vi "诊断标定3 - 副本.vi"(8 "CAN端口":u16(ring), 9 "设备索引号":u16(ring), 10 "CAN卡类型":u32(ring)=21) -> ()   [LabVIEW 2013] (continued)
            n1767 = property on="最小允许单体电压" class="DigNum (严格)"("Disabled"=w2295) -> ()  [unwired: 2 in, 2 out]
            n1768 = property on="电流步长" class="DigNum (严格)"("Disabled"=w2295) -> ()  [unwired: 2 in, 2 out]
            n1769 = property on="SOC" class="DigNum (严格)"("Disabled"=w2295) -> ()  [unwired: 2 in, 2 out]
            n1770 = property on="充电总安时" class="DigNum (严格)"("Disabled"=w2291) -> ()  [unwired: 2 in, 2 out]
            n1771 = property on="放电总安时" class="DigNum (严格)"("Disabled"=w2291) -> ()  [unwired: 2 in, 2 out]
            n1772 = Not(x=w2284) -> (.not. x?=w2299:bool)
            n1773 = global read "功能码全局.vi" "24"() -> (w2289:bool[])
            n1774 = global read "功能码全局.vi" "23"() -> (w2290:bool[])
            n1775 = Index Array(array=w2289) -> (element #7=w2287:bool)  [unwired: 8 in, 7 out]
            n1776 = Index Array(array=w2290) -> (element #7=w2288:bool)  [unwired: 8 in, 7 out]
          }
          frame "充电次数" {
            w2304 = 2
            w2313 = 2
            w2314 = 2
            w2305 = 2
            w2315 = 2
            w2301 = FALSE ("1 6")
            n1777 = property on="串联数" class="DigNum (严格)"("Disabled"=w2315) -> ()  [unwired: 2 in, 2 out]
            n1778 = property on="并联数" class="DigNum (严格)"("Disabled"=w2315) -> ()  [unwired: 2 in, 2 out]
            n1779 = property on="电池厂家" class="DigNum (严格)"("Disabled"=w2315) -> ()  [unwired: 2 in, 2 out]
            n1780 = property on="电池类型" class="DigNum (严格)"("Disabled"=w2315) -> ()  [unwired: 2 in, 2 out]
            n1781 = property on="额定能量" class="DigNum (严格)"("Disabled"=w2315) -> ()  [unwired: 2 in, 2 out]
            n1782 = property on="额定容量" class="DigNum (严格)"("Disabled"=w2315) -> ()  [unwired: 2 in, 2 out]
            n1783 = property on="实际容量" class="DigNum (严格)"("Disabled"=w2315) -> ()  [unwired: 2 in, 2 out]
            n1784 = Select(t=0, s=w2310, f=1) -> (s? t:f=w2302:i32)
            n1785 = property on="生产日期" class="Str"("DisabledEnum"=w2304) -> ()  [unwired: 2 in, 2 out]
            n1786 = property on="电池包序号" class="DigNum (严格)"("DisabledEnum"=w2304) -> ()  [unwired: 2 in, 2 out]
            n1787 = property on="车牌号" class="Str"("DisabledEnum"=w2304) -> ()  [unwired: 2 in, 2 out]
            n1788 = property on="电池组信息" class="Clust (严格)"("Disabled"=w2302) -> ()  [unwired: 2 in, 2 out]
            n1789 = property on="电池包组号" class="DigNum (严格)"("DisabledEnum"=w2304) -> ()  [unwired: 2 in, 2 out]
            n1790 = property on="额定总压" class="DigNum (严格)"("Disabled"=w2305) -> ()  [unwired: 2 in, 2 out]
            n1791 = property on="产权标识" class="DigNum (严格)"("Disabled"=w2305) -> ()  [unwired: 2 in, 2 out]
            n1792 = property on="应用车型" class="DigNum (严格)"("Disabled"=w2305) -> ()  [unwired: 2 in, 2 out]
            n1793 = property on="放空次数" class="DigNum (严格)"("DisabledEnum"=w2302) -> (error out=w2303:errorcluster)  [unwired: 2 in, 1 out]
            n1794 = property on="充满次数" class="DigNum (严格)"("DisabledEnum"=w2302) -> ()  [unwired: 2 in, 2 out]
            n1795 = property on="充电次数" class="DigNum (严格)"("DisabledEnum"=w2302) -> ()  [unwired: 2 in, 2 out]
            n1796 = property on="最大允许单体电压" class="DigNum (严格)"("Disabled"=w2314) -> ()  [unwired: 2 in, 2 out]
            n1797 = property on="最大允许总电压" class="DigNum (严格)"("Disabled"=w2314) -> ()  [unwired: 2 in, 2 out]
            n1798 = property on="最大允许温度" class="DigNum (严格)"("Disabled"=w2314) -> ()  [unwired: 2 in, 2 out]
            n1799 = property on="最小允许温度" class="DigNum (严格)"("Disabled"=w2314) -> ()  [unwired: 2 in, 2 out]
            n1800 = property on="最大允许充电电流" class="DigNum (严格)"("Disabled"=w2314) -> ()  [unwired: 2 in, 2 out]
            n1801 = property on="最小允许充电电流" class="DigNum (严格)"(error in=w2303, "Disabled"=w2314) -> ()  [unwired: 1 in, 2 out]
            n1802 = property on="最小允许单体电压" class="DigNum (严格)"("Disabled"=w2314) -> ()  [unwired: 2 in, 2 out]
            n1803 = property on="电流步长" class="DigNum (严格)"("Disabled"=w2314) -> ()  [unwired: 2 in, 2 out]
            n1804 = property on="SOC" class="DigNum (严格)"("Disabled"=w2314) -> ()  [unwired: 2 in, 2 out]
            n1805 = property on="充电总安时" class="DigNum (严格)"("Disabled"=w2313) -> ()  [unwired: 2 in, 2 out]
            n1806 = property on="放电总安时" class="DigNum (严格)"("Disabled"=w2313) -> ()  [unwired: 2 in, 2 out]
            n1807 = Not(x=w2301) -> (.not. x?=w2316:bool)
            n1808 = global read "功能码全局.vi" "24"() -> (w2308:bool[])
            n1809 = global read "功能码全局.vi" "23"() -> (w2309:bool[])
            n1810 = Index Array(array=w2308) -> (element #8=w2307:bool)  [unwired: 8 in, 7 out]
            n1811 = Index Array(array=w2309) -> (element #8=w2306:bool)  [unwired: 8 in, 7 out]
          }
          frame "SOC" {
            w2320 = 2
            w2319 = 2
            w2329 = 2
            w2330 = 2
            w2331 = 2
            w2333 = 2
            w2318 = FALSE ("1 6")
            n1812 = property on="串联数" class="DigNum (严格)"("Disabled"=w2333) -> ()  [unwired: 2 in, 2 out]
            n1813 = property on="并联数" class="DigNum (严格)"("Disabled"=w2333) -> ()  [unwired: 2 in, 2 out]
            n1814 = property on="电池厂家" class="DigNum (严格)"("Disabled"=w2333) -> ()  [unwired: 2 in, 2 out]
            n1815 = property on="电池类型" class="DigNum (严格)"("Disabled"=w2333) -> ()  [unwired: 2 in, 2 out]
            n1816 = property on="额定能量" class="DigNum (严格)"("Disabled"=w2333) -> ()  [unwired: 2 in, 2 out]
            n1817 = property on="额定容量" class="DigNum (严格)"("Disabled"=w2333) -> ()  [unwired: 2 in, 2 out]
            n1818 = property on="实际容量" class="DigNum (严格)"("Disabled"=w2333) -> ()  [unwired: 2 in, 2 out]
            n1819 = Select(t=0, s=w2326, f=1) -> (s? t:f=w2325:i32)
            n1820 = property on="生产日期" class="Str"("DisabledEnum"=w2320) -> ()  [unwired: 2 in, 2 out]
            n1821 = property on="电池包序号" class="DigNum (严格)"("DisabledEnum"=w2320) -> ()  [unwired: 2 in, 2 out]
            n1822 = property on="车牌号" class="Str"("DisabledEnum"=w2320) -> ()  [unwired: 2 in, 2 out]
            n1823 = property on="电池包组号" class="DigNum (严格)"("DisabledEnum"=w2320) -> ()  [unwired: 2 in, 2 out]
            n1824 = property on="电池组信息" class="Clust (严格)"("Disabled"=w2325) -> ()  [unwired: 2 in, 2 out]
            n1825 = property on="SOC" class="DigNum (严格)"("Disabled"=w2325) -> ()  [unwired: 2 in, 2 out]
            n1826 = property on="额定总压" class="DigNum (严格)"("Disabled"=2) -> ()  [unwired: 2 in, 2 out]
            n1827 = property on="产权标识" class="DigNum (严格)"("Disabled"=w2331) -> ()  [unwired: 2 in, 2 out]
            n1828 = property on="应用车型" class="DigNum (严格)"("Disabled"=w2331) -> ()  [unwired: 2 in, 2 out]
            n1829 = property on="放空次数" class="DigNum (严格)"("DisabledEnum"=w2319) -> ()  [unwired: 2 in, 2 out]
            n1830 = property on="充满次数" class="DigNum (严格)"("DisabledEnum"=w2319) -> ()  [unwired: 2 in, 2 out]
            n1831 = property on="充电次数" class="DigNum (严格)"("DisabledEnum"=w2319) -> ()  [unwired: 2 in, 2 out]
            n1832 = property on="最大允许单体电压" class="DigNum (严格)"("Disabled"=w2330) -> ()  [unwired: 2 in, 2 out]
            n1833 = property on="最大允许总电压" class="DigNum (严格)"("Disabled"=w2330) -> ()  [unwired: 2 in, 2 out]
            n1834 = property on="最大允许温度" class="DigNum (严格)"("Disabled"=w2330) -> ()  [unwired: 2 in, 2 out]
            n1835 = property on="最小允许温度" class="DigNum (严格)"("Disabled"=w2330) -> ()  [unwired: 2 in, 2 out]
            n1836 = property on="最大允许充电电流" class="DigNum (严格)"("Disabled"=w2330) -> ()  [unwired: 2 in, 2 out]
            n1837 = property on="最小允许充电电流" class="DigNum (严格)"("Disabled"=w2330) -> ()  [unwired: 2 in, 2 out]
            n1838 = property on="最小允许单体电压" class="DigNum (严格)"("Disabled"=w2330) -> ()  [unwired: 2 in, 2 out]
            n1839 = property on="电流步长" class="DigNum (严格)"("Disabled"=w2330) -> ()  [unwired: 2 in, 2 out]
            n1840 = property on="充电总安时" class="DigNum (严格)"("Disabled"=w2329) -> ()  [unwired: 2 in, 2 out]
            n1841 = property on="放电总安时" class="DigNum (严格)"("Disabled"=w2329) -> ()  [unwired: 2 in, 2 out]
            n1842 = Not(x=w2318) -> (.not. x?=w2334:bool)
            n1843 = global read "功能码全局.vi" "24"() -> (w2323:bool[])
            n1844 = global read "功能码全局.vi" "23"() -> (w2324:bool[])
            n1845 = Index Array(array=w2323) -> (element #6=w2322:bool)  [unwired: 8 in, 7 out]
            n1846 = Index Array(array=w2324) -> (element #6=w2321:bool)  [unwired: 8 in, 7 out]
          }
          frame "车牌号" {
            w2339 = 2
            w2338 = 2
            w2348 = 2
            w2349 = 2
            w2350 = 2
            w2352 = 2
            w2336 = FALSE ("1 6")
            n1847 = property on="串联数" class="DigNum (严格)"("Disabled"=w2352) -> ()  [unwired: 2 in, 2 out]
            n1848 = property on="并联数" class="DigNum (严格)"("Disabled"=w2352) -> ()  [unwired: 2 in, 2 out]
            n1849 = property on="电池厂家" class="DigNum (严格)"("Disabled"=w2352) -> ()  [unwired: 2 in, 2 out]
            n1850 = property on="电池类型" class="DigNum (严格)"("Disabled"=w2352) -> ()  [unwired: 2 in, 2 out]
            n1851 = property on="额定能量" class="DigNum (严格)"("Disabled"=w2352) -> ()  [unwired: 2 in, 2 out]
            n1852 = property on="额定容量" class="DigNum (严格)"("Disabled"=w2352) -> ()  [unwired: 2 in, 2 out]
            n1853 = property on="实际容量" class="DigNum (严格)"("Disabled"=w2352) -> ()  [unwired: 2 in, 2 out]
            n1854 = Select(t=0, s=w2344, f=1) -> (s? t:f=w2337:i32)
            n1855 = property on="生产日期" class="Str"("DisabledEnum"=w2339) -> ()  [unwired: 2 in, 2 out]
            n1856 = property on="电池包序号" class="DigNum (严格)"("DisabledEnum"=w2339) -> ()  [unwired: 2 in, 2 out]
            n1857 = property on="电池包组号" class="DigNum (严格)"("DisabledEnum"=w2339) -> ()  [unwired: 2 in, 2 out]
            n1858 = property on="电池组信息" class="Clust (严格)"("Disabled"=w2337) -> ()  [unwired: 2 in, 2 out]
            n1859 = property on="车牌号" class="Str"("DisabledEnum"=w2337) -> ()  [unwired: 2 in, 2 out]
            n1860 = property on="额定总压" class="DigNum (严格)"("Disabled"=2) -> ()  [unwired: 2 in, 2 out]
            n1861 = property on="产权标识" class="DigNum (严格)"("Disabled"=w2350) -> ()  [unwired: 2 in, 2 out]
            n1862 = property on="应用车型" class="DigNum (严格)"("Disabled"=w2350) -> ()  [unwired: 2 in, 2 out]
            n1863 = property on="放空次数" class="DigNum (严格)"("DisabledEnum"=w2338) -> ()  [unwired: 2 in, 2 out]
            n1864 = property on="充满次数" class="DigNum (严格)"("DisabledEnum"=w2338) -> ()  [unwired: 2 in, 2 out]
            n1865 = property on="充电次数" class="DigNum (严格)"("DisabledEnum"=w2338) -> ()  [unwired: 2 in, 2 out]
            n1866 = property on="最大允许单体电压" class="DigNum (严格)"("Disabled"=w2349) -> ()  [unwired: 2 in, 2 out]
            n1867 = property on="最大允许总电压" class="DigNum (严格)"("Disabled"=w2349) -> ()  [unwired: 2 in, 2 out]
            n1868 = property on="最大允许温度" class="DigNum (严格)"("Disabled"=w2349) -> ()  [unwired: 2 in, 2 out]
            n1869 = property on="最小允许温度" class="DigNum (严格)"("Disabled"=w2349) -> ()  [unwired: 2 in, 2 out]
            n1870 = property on="最大允许充电电流" class="DigNum (严格)"("Disabled"=w2349) -> ()  [unwired: 2 in, 2 out]
            n1871 = property on="最小允许充电电流" class="DigNum (严格)"("Disabled"=w2349) -> ()  [unwired: 2 in, 2 out]
            n1872 = property on="最小允许单体电压" class="DigNum (严格)"("Disabled"=w2349) -> ()  [unwired: 2 in, 2 out]
            n1873 = property on="电流步长" class="DigNum (严格)"("Disabled"=w2349) -> ()  [unwired: 2 in, 2 out]
            n1874 = property on="SOC" class="DigNum (严格)"("Disabled"=2) -> ()  [unwired: 2 in, 2 out]
            n1875 = property on="充电总安时" class="DigNum (严格)"("Disabled"=w2348) -> ()  [unwired: 2 in, 2 out]
            n1876 = property on="放电总安时" class="DigNum (严格)"("Disabled"=w2348) -> ()  [unwired: 2 in, 2 out]
            n1877 = Not(x=w2336) -> (.not. x?=w2353:bool)
            n1878 = global read "功能码全局.vi" "24"() -> (w2342:bool[])
            n1879 = global read "功能码全局.vi" "23"() -> (w2343:bool[])
            n1880 = Index Array(array=w2342) -> (element #5=w2340:bool)  [unwired: 8 in, 7 out]
            n1881 = Index Array(array=w2343) -> (element #5=w2341:bool)  [unwired: 8 in, 7 out]
          }
          frame "充电参数" {
            w2357 = 2
            w2356 = 2
            w2366 = 2
            w2367 = 2
            w2369 = 2
            w2355 = FALSE ("1 6")
            n1882 = property on="串联数" class="DigNum (严格)"("Disabled"=w2369) -> ()  [unwired: 2 in, 2 out]
            n1883 = property on="并联数" class="DigNum (严格)"("Disabled"=w2369) -> ()  [unwired: 2 in, 2 out]
            n1884 = property on="电池厂家" class="DigNum (严格)"("Disabled"=w2369) -> ()  [unwired: 2 in, 2 out]
            n1885 = property on="电池类型" class="DigNum (严格)"("Disabled"=w2369) -> ()  [unwired: 2 in, 2 out]
            n1886 = property on="额定能量" class="DigNum (严格)"("Disabled"=w2369) -> ()  [unwired: 2 in, 2 out]
            n1887 = property on="额定容量" class="DigNum (严格)"("Disabled"=w2369) -> ()  [unwired: 2 in, 2 out]
            n1888 = property on="实际容量" class="DigNum (严格)"("Disabled"=w2369) -> ()  [unwired: 2 in, 2 out]
            n1889 = Select(t=0, s=w2363, f=1) -> (s? t:f=w2362:i32)
            n1890 = property on="生产日期" class="Str"("DisabledEnum"=w2357) -> ()  [unwired: 2 in, 2 out]
            n1891 = property on="电池包序号" class="DigNum (严格)"("DisabledEnum"=w2357) -> ()  [unwired: 2 in, 2 out]
            n1892 = property on="车牌号" class="Str"("DisabledEnum"=w2357) -> ()  [unwired: 2 in, 2 out]
            n1893 = property on="电池组信息" class="Clust (严格)"("Disabled"=w2362) -> ()  [unwired: 2 in, 2 out]
            n1894 = property on="电池包组号" class="DigNum (严格)"("DisabledEnum"=w2357) -> ()  [unwired: 2 in, 2 out]
            n1895 = property on="额定总压" class="DigNum (严格)"("Disabled"=2) -> ()  [unwired: 2 in, 2 out]
            n1896 = property on="产权标识" class="DigNum (严格)"("Disabled"=w2367) -> ()  [unwired: 2 in, 2 out]
            n1897 = property on="应用车型" class="DigNum (严格)"("Disabled"=w2367) -> ()  [unwired: 2 in, 2 out]
            n1898 = property on="放空次数" class="DigNum (严格)"("DisabledEnum"=w2356) -> ()  [unwired: 2 in, 2 out]
            n1899 = property on="充满次数" class="DigNum (严格)"("DisabledEnum"=w2356) -> ()  [unwired: 2 in, 2 out]
            n1900 = property on="充电次数" class="DigNum (严格)"("DisabledEnum"=w2356) -> ()  [unwired: 2 in, 2 out]
            n1901 = property on="最大允许单体电压" class="DigNum (严格)"("Disabled"=w2362) -> ()  [unwired: 2 in, 2 out]
            n1902 = property on="最大允许总电压" class="DigNum (严格)"("Disabled"=w2362) -> ()  [unwired: 2 in, 2 out]
            n1903 = property on="最大允许温度" class="DigNum (严格)"("Disabled"=w2362) -> ()  [unwired: 2 in, 2 out]
            n1904 = property on="最小允许温度" class="DigNum (严格)"("Disabled"=w2362) -> ()  [unwired: 2 in, 2 out]
            n1905 = property on="最大允许充电电流" class="DigNum (严格)"("Disabled"=w2362) -> ()  [unwired: 2 in, 2 out]
            n1906 = property on="最小允许充电电流" class="DigNum (严格)"("Disabled"=w2362) -> ()  [unwired: 2 in, 2 out]
            n1907 = property on="最小允许单体电压" class="DigNum (严格)"("Disabled"=w2362) -> ()  [unwired: 2 in, 2 out]
            n1908 = property on="电流步长" class="DigNum (严格)"("Disabled"=w2362) -> ()  [unwired: 2 in, 2 out]
            n1909 = property on="SOC" class="DigNum (严格)"("Disabled"=w2366) -> ()  [unwired: 2 in, 2 out]
            n1910 = property on="充电总安时" class="DigNum (严格)"("Disabled"=w2366) -> ()  [unwired: 2 in, 2 out]
            n1911 = property on="放电总安时" class="DigNum (严格)"("Disabled"=w2366) -> ()  [unwired: 2 in, 2 out]
            n1912 = Not(x=w2355) -> (.not. x?=w2370:bool)
            n1913 = global read "功能码全局.vi" "24"() -> (w2360:bool[])
            n1914 = global read "功能码全局.vi" "23"() -> (w2361:bool[])
            n1915 = Index Array(array=w2360) -> (element #4=w2358:bool)  [unwired: 8 in, 7 out]
            n1916 = Index Array(array=w2361) -> (element #4=w2359:bool)  [unwired: 8 in, 7 out]
          }
          frame "均衡参数" {
            w2372 = FALSE ("1 6")
            n1917 = Select(t=0, s=w2378, f=1) -> (s? t:f=w2376:i32)
            n1918 = property on="均衡计算-电压高阀值1级" class="DigNum (严格)"("DisabledEnum"=w2376) -> ()  [unwired: 2 in, 2 out]
            n1919 = property on="均衡计算-电压高阀值2级" class="DigNum (严格)"("DisabledEnum"=w2376) -> ()  [unwired: 2 in, 2 out]
            n1920 = property on="均衡计算-电压低阀值1级" class="DigNum (严格)"("DisabledEnum"=w2376) -> ()  [unwired: 2 in, 2 out]
            n1921 = property on="均衡计算-电压低阀值2级" class="DigNum (严格)"("DisabledEnum"=w2376) -> ()  [unwired: 2 in, 2 out]
            n1922 = property on="均衡计算-最低电压阀值" class="DigNum (严格)"("DisabledEnum"=w2376) -> ()  [unwired: 2 in, 2 out]
            n1923 = property on="均衡停止-最低电压阀值" class="DigNum (严格)"("DisabledEnum"=w2376) -> ()  [unwired: 2 in, 2 out]
            n1924 = property on="均衡计算-电压极差阀值" class="DigNum (严格)"("DisabledEnum"=w2376) -> ()  [unwired: 2 in, 2 out]
            n1925 = property on="均衡参数" class="Clust (严格)"("DisabledEnum"=w2376) -> ()  [unwired: 2 in, 2 out]
            n1926 = property on="充电结束电压(90%)" class="DigNum (严格)"("DisabledEnum"=w2376) -> ()  [unwired: 2 in, 2 out]
            n1927 = property on="充电结束电压(91%)" class="DigNum (严格)"("DisabledEnum"=w2376) -> ()  [unwired: 2 in, 2 out]
            n1928 = property on="充电结束电压(92%)" class="DigNum (严格)"("DisabledEnum"=w2376) -> ()  [unwired: 2 in, 2 out]
            n1929 = property on="充电结束电压(93%)" class="DigNum (严格)"("DisabledEnum"=w2376) -> ()  [unwired: 2 in, 2 out]
            n1930 = property on="充电结束电压(94%)" class="DigNum (严格)"("DisabledEnum"=w2376) -> ()  [unwired: 2 in, 2 out]
            n1931 = property on="充电结束电压(95%)" class="DigNum (严格)"("DisabledEnum"=w2376) -> ()  [unwired: 2 in, 2 out]
            n1932 = property on="充电结束电压(96%)" class="DigNum (严格)"("DisabledEnum"=w2376) -> ()  [unwired: 2 in, 2 out]
            n1933 = property on="充电结束电压(97%)" class="DigNum (严格)"("DisabledEnum"=w2376) -> ()  [unwired: 2 in, 2 out]
            n1934 = property on="充电结束电压(98%)" class="DigNum (严格)"("DisabledEnum"=w2376) -> ()  [unwired: 2 in, 2 out]
            n1935 = property on="充电结束电压(99%)" class="DigNum (严格)"("DisabledEnum"=w2376) -> ()  [unwired: 2 in, 2 out]
            n1936 = property on="充电结束电压(100%)" class="DigNum (严格)"("DisabledEnum"=w2376) -> ()  [unwired: 2 in, 2 out]
            n1937 = disable-structure shown="启用" {
              disable-tunnel: [w2382 w2384] -> w2375
              disable-tunnel: [w2381 w2384] -> w2374
              frame Enabled {
                n1938 = global read "功能码全局.vi" "18"() -> (w2383:bool[])
                n1939 = Index Array(array=w2383) -> (element #1=w2382:bool, element #2=w2381:bool)  [unwired: 8 in, 6 out]
              }
              frame Disabled {
                w2384 = TRUE
              }
            }
            n1940 = Not(x=w2372) -> (.not. x?=w2373:bool)
          }
          frame "均衡阀值" {
            w2387 = 2
            w2385 = FALSE ("1 6")
            n1941 = Select(t=0, s=w2392, f=1) -> (s? t:f=w2390:i32)
            n1942 = property on="均衡计算-电压高阀值1级" class="DigNum (严格)"("DisabledEnum"=w2390) -> ()  [unwired: 2 in, 2 out]
            n1943 = property on="均衡计算-电压高阀值2级" class="DigNum (严格)"("DisabledEnum"=w2390) -> ()  [unwired: 2 in, 2 out]
            n1944 = property on="均衡计算-电压低阀值1级" class="DigNum (严格)"("DisabledEnum"=w2390) -> ()  [unwired: 2 in, 2 out]
            n1945 = property on="均衡计算-电压低阀值2级" class="DigNum (严格)"("DisabledEnum"=w2390) -> ()  [unwired: 2 in, 2 out]
            n1946 = property on="均衡计算-最低电压阀值" class="DigNum (严格)"("DisabledEnum"=w2390) -> ()  [unwired: 2 in, 2 out]
            n1947 = property on="均衡停止-最低电压阀值" class="DigNum (严格)"("DisabledEnum"=w2390) -> ()  [unwired: 2 in, 2 out]
            n1948 = property on="均衡计算-电压极差阀值" class="DigNum (严格)"("DisabledEnum"=w2390) -> ()  [unwired: 2 in, 2 out]
            n1949 = property on="均衡参数" class="Clust (严格)"("DisabledEnum"=w2390) -> ()  [unwired: 2 in, 2 out]
            n1950 = property on="充电结束电压(90%)" class="DigNum (严格)"("DisabledEnum"=w2387) -> ()  [unwired: 2 in, 2 out]
            n1951 = property on="充电结束电压(91%)" class="DigNum (严格)"("DisabledEnum"=w2387) -> ()  [unwired: 2 in, 2 out]
            n1952 = property on="充电结束电压(92%)" class="DigNum (严格)"("DisabledEnum"=w2387) -> ()  [unwired: 2 in, 2 out]
            n1953 = property on="充电结束电压(93%)" class="DigNum (严格)"("DisabledEnum"=w2387) -> ()  [unwired: 2 in, 2 out]
            n1954 = property on="充电结束电压(94%)" class="DigNum (严格)"("DisabledEnum"=w2387) -> ()  [unwired: 2 in, 2 out]
            n1955 = property on="充电结束电压(95%)" class="DigNum (严格)"("DisabledEnum"=w2387) -> ()  [unwired: 2 in, 2 out]
            n1956 = property on="充电结束电压(96%)" class="DigNum (严格)"("DisabledEnum"=w2387) -> ()  [unwired: 2 in, 2 out]
            n1957 = property on="充电结束电压(97%)" class="DigNum (严格)"("DisabledEnum"=w2387) -> ()  [unwired: 2 in, 2 out]
            n1958 = property on="充电结束电压(98%)" class="DigNum (严格)"("DisabledEnum"=w2387) -> ()  [unwired: 2 in, 2 out]
            n1959 = property on="充电结束电压(99%)" class="DigNum (严格)"("DisabledEnum"=w2387) -> ()  [unwired: 2 in, 2 out]
            n1960 = property on="充电结束电压(100%)" class="DigNum (严格)"("DisabledEnum"=w2387) -> ()  [unwired: 2 in, 2 out]
            n1961 = disable-structure shown="启用" {
              disable-tunnel: [w2396 w2398] -> w2389
              disable-tunnel: [w2395 w2398] -> w2388
              frame Enabled {
                n1962 = global read "功能码全局.vi" "18"() -> (w2397:bool[])
                n1963 = Index Array(array=w2397) -> (element #1=w2396:bool, element #2=w2395:bool)  [unwired: 8 in, 6 out]
              }
              frame Disabled {
                w2398 = TRUE
              }
            }
            n1964 = Not(x=w2385) -> (.not. x?=w2386:bool)
          }
          frame "充电结束电压" {
            w2402 = 2
            w2399 = FALSE ("1 6")
            n1965 = Select(t=0, s=w2406, f=1) -> (s? t:f=w2401:i32)
            n1966 = property on="均衡计算-电压高阀值1级" class="DigNum (严格)"("DisabledEnum"=w2402) -> ()  [unwired: 2 in, 2 out]
            n1967 = property on="均衡计算-电压高阀值2级" class="DigNum (严格)"("DisabledEnum"=w2402) -> ()  [unwired: 2 in, 2 out]
            n1968 = property on="均衡计算-电压低阀值1级" class="DigNum (严格)"("DisabledEnum"=w2402) -> ()  [unwired: 2 in, 2 out]
            n1969 = property on="均衡计算-电压低阀值2级" class="DigNum (严格)"("DisabledEnum"=w2402) -> ()  [unwired: 2 in, 2 out]
            n1970 = property on="均衡计算-最低电压阀值" class="DigNum (严格)"("DisabledEnum"=w2402) -> ()  [unwired: 2 in, 2 out]
            n1971 = property on="均衡停止-最低电压阀值" class="DigNum (严格)"("DisabledEnum"=w2402) -> ()  [unwired: 2 in, 2 out]
            n1972 = property on="均衡计算-电压极差阀值" class="DigNum (严格)"("DisabledEnum"=w2402) -> ()  [unwired: 2 in, 2 out]
            n1973 = property on="均衡参数" class="Clust (严格)"("DisabledEnum"=w2401) -> ()  [unwired: 2 in, 2 out]
            n1974 = property on="充电结束电压(90%)" class="DigNum (严格)"("DisabledEnum"=w2401) -> ()  [unwired: 2 in, 2 out]
            n1975 = property on="充电结束电压(91%)" class="DigNum (严格)"("DisabledEnum"=w2401) -> ()  [unwired: 2 in, 2 out]
            n1976 = property on="充电结束电压(92%)" class="DigNum (严格)"("DisabledEnum"=w2401) -> ()  [unwired: 2 in, 2 out]
            n1977 = property on="充电结束电压(93%)" class="DigNum (严格)"("DisabledEnum"=w2401) -> ()  [unwired: 2 in, 2 out]
            n1978 = property on="充电结束电压(94%)" class="DigNum (严格)"("DisabledEnum"=w2401) -> ()  [unwired: 2 in, 2 out]
            n1979 = property on="充电结束电压(95%)" class="DigNum (严格)"("DisabledEnum"=w2401) -> ()  [unwired: 2 in, 2 out]
            n1980 = property on="充电结束电压(96%)" class="DigNum (严格)"("DisabledEnum"=w2401) -> ()  [unwired: 2 in, 2 out]
            n1981 = property on="充电结束电压(97%)" class="DigNum (严格)"("DisabledEnum"=w2401) -> ()  [unwired: 2 in, 2 out]
            n1982 = property on="充电结束电压(98%)" class="DigNum (严格)"("DisabledEnum"=w2401) -> ()  [unwired: 2 in, 2 out]
            n1983 = property on="充电结束电压(99%)" class="DigNum (严格)"("DisabledEnum"=w2401) -> ()  [unwired: 2 in, 2 out]
            n1984 = property on="充电结束电压(100%)" class="DigNum (严格)"("DisabledEnum"=w2401) -> ()  [unwired: 2 in, 2 out]
            n1985 = disable-structure shown="启用" {
              disable-tunnel: [w2410 w2412] -> w2404
              disable-tunnel: [w2409 w2412] -> w2403
              frame Enabled {
                n1986 = global read "功能码全局.vi" "18"() -> (w2411:bool[])
                n1987 = Index Array(array=w2411) -> (element #1=w2410:bool, element #2=w2409:bool)  [unwired: 8 in, 6 out]
              }
              frame Disabled {
                w2412 = TRUE
              }
            }
            n1988 = Not(x=w2399) -> (.not. x?=w2400:bool)
          }
          frame "假", Default {
            w2413 = FALSE ("1 6")
            n1989 = Not(x=w2413) -> (.not. x?=w2414:bool)
          }
        }
        n1990 = local write "等级 2"(w1994) -> ()
        n1991 = local write "1 6"(w1993) -> ()
        n1992 = local write "1 7"(w1992) -> ()
        n1993 = local write "1 8"(w1991) -> ()
        n1994 = local write "1 9"(w1990) -> ()
        n1995 = local write "1 10"(w1989) -> ()
        n1996 = local write "1 12"(w1983) -> ()
        n1997 = property on="单个读取" class="Bool (严格)"("Visible"=w1988) -> ()  [unwired: 2 in, 2 out]
        n1998 = property on="单个写入" class="Bool (严格)"("Visible"=w1987) -> ()  [unwired: 2 in, 2 out]
      }
      event "从板个数": Value Change {
        n1999 = event-data() -> ()  [unwired: 7 out]
        n2000 = local read "从板个数"() -> (w2416:dbl)
        n2001 = call "多从板对应参数-new.vi"("从板个数"=w2416) -> ("输出数组"=w2417:string[])  [unwired: 1 in]
        n2002 = control-ref of="项目信息"() -> (w2418:refnum<vi>)
        n2003 = stacked-sequence {
          tunnel: w2418 -> [_ w2425 w2429]
          tunnel: w2417 -> [_ w2424 w2428]
          frame #0 {
            n2004 = local write "项目信息"(string[][] [] ("项目信息")) -> ()
          }
          frame #1 {
            n2005 = call "表格数据输入-8.6.vi"("行数"=u32 0, "列数"=u32 0, "字符串数组"=w2424, "表格引用"=w2425) -> ()  [unwired: 8 out]
          }
          frame #2 {
            n2006 = Array Size(array=w2428) -> (size(s)=w2427:i32)
            n2007 = for {
              N: w2427 -> [_]
              tunnel: [""] -> w2426 mode=indexing
            }
            n2008 = call "表格数据输入-8.6.vi"("行数"=u32 0, "列数"=u32 1, "字符串数组"=w2426, "表格引用"=w2429) -> ()  [unwired: 8 out]
          }
        }
      }
      event "主界面选项": Value Change {
        n2009 = event-data() -> ("NewVal"=w2433:enum32{"单选选项1", "单选选项2", "单选选项2 2", "单选选项2 3"})  [unwired: 6 out]
        n2010 = control-ref of="单选选项2 2"() -> (w2438:refnum<vi>)
        n2011 = control-ref of="单选选项2"() -> (w2440:refnum<vi>)
        n2012 = control-ref of="单选选项1"() -> (w2439:refnum<vi>)
        n2013 = control-ref of="单选选项2 3"() -> (w2434:refnum<vi>)
        n2014 = Build Array(w2439, w2440, w2438, w2434) -> (w2437:refnum<vi>[])
        n2015 = case shown="\"单选选项2 3\"" w2433 {
          selector: w2433 -> [w2451 w2456 w2461 w2466]
          tunnel: w2437 -> [w2452 w2457 w2462 w2467]
          tunnel: [w2450 w2455 w2460 w2465] -> w2443
          tunnel: [w2449 w2454 w2459 w2464] -> w2442
          tunnel: [enum32{"读写参数", "版本读取", "其它诊断"}."读写参数" ("选项卡控件 2") enum32{"读写参数", "版本读取", "其它诊断"}."版本读取" ("选项卡控件 2") enum32{"读写参数", "版本读取", "其它诊断"}."其它诊断" ("选项卡控件 2") enum32{"读写参数", "版本读取", "其它诊断", "高压板校正"}."高压板校正" ("选项卡控件 2")] -> w2441
          frame "单选选项1", Default {
            n2016 = Delete From Array(array=w2452, index=w2451) -> (deleted portion=w2449:refnum<vi>, array with subset deleted=w2450:refnum<vi>[])  [unwired: 1 in]
          }
          frame "单选选项2" {
            n2017 = Delete From Array(array=w2457, index=w2456) -> (deleted portion=w2454:refnum<vi>, array with subset deleted=w2455:refnum<vi>[])  [unwired: 1 in]
          }
          frame "单选选项2 2" {
            n2018 = Delete From Array(array=w2462, index=w2461) -> (deleted portion=w2459:refnum<vi>, array with subset deleted=w2460:refnum<vi>[])  [unwired: 1 in]
          }
          frame "单选选项2 3" {
            n2019 = Delete From Array(array=w2467, index=w2466) -> (deleted portion=w2464:refnum<vi>, array with subset deleted=w2465:refnum<vi>[])  [unwired: 1 in]
          }
        }
        n2020 = local write "面板选择"(w2441) -> ()
        n2021 = for {
          tunnel: u32 16777215 -> [w2447]
          tunnel: w2443 -> [w2446] mode=indexing
          n2022 = property class="Bool (严格)"(reference=w2446, "BoolText.TextColor"=w2447) -> ()  [unwired: 1 in, 2 out]
        }
        n2023 = property class="Bool (严格)"(reference=w2442, "BoolText.TextColor"=u32 65511) -> ()  [unwired: 1 in, 2 out]
      }
      event "主从板": Value Change {
        w2469 = FALSE ("可见")
        n2024 = event-data() -> ()  [unwired: 7 out]
        n2025 = control-ref of="单选选项2"() -> (w2477:refnum<vi>)
        n2026 = control-ref of="单选选项1"() -> (w2476:refnum<vi>)
        n2027 = local read "主从板"() -> (w2484:enum32{"单选选项2", "单选选项1"})
        n2028 = Build Array(w2477, w2476) -> (w2483:refnum<vi>[])
        n2029 = case shown="\"单选选项2\"" w2484 {
          selector: w2484 -> [w2529 w2572]
          tunnel: w2483 -> [w2530 w2571]
          tunnel: [enum32{"主板", "从板"}."主板" ("主从选择") enum32{"主板", "从板"}."从板" ("主从选择")] -> w2482
          tunnel: [w2528 w2570] -> w2479
          tunnel: [w2527 w2569] -> w2478
          tunnel: [TRUE FALSE] -> w2474
          tunnel: [w2488 w2549] -> w2471
          tunnel: [w2489 w2554] -> w2470
          tunnel: [FALSE ("可见") TRUE ("可见")] -> w2468
          frame "单选选项1", Default {
            n2030 = global read "功能码全局.vi" "主板项目信息7"() -> (w2500:bool[])
            n2031 = global read "功能码全局.vi" "主板项目信息4"() -> (w2523:bool[])
            n2032 = global read "功能码全局.vi" "主板控制类信息10"() -> (w2504:bool[])
            n2033 = global read "功能码全局.vi" "主板故障阀值9"() -> (w2501:bool[])
            n2034 = global read "功能码全局.vi" "主板项目信息5"() -> (w2514:bool[])
            n2035 = global read "功能码全局.vi" "主板项目信息6"() -> (w2524:bool[])
            n2036 = global read "功能码全局.vi" "主板版本号11"() -> (w2515:bool[])
            n2037 = Delete From Array(array=w2524, length=1 ("长度"), index=0 ("索引")) -> (deleted portion=w2513:bool[], array with subset deleted=w2496:bool[])
            n2038 = Index Array(array=w2523, index #1=5 ("索引"), index #2=6 ("索引")) -> (element #1=w2512:bool, element #2=w2495:bool)
            n2039 = Index Array(array=w2515) -> (element #1=w2508:bool, element #2=w2491:bool)  [unwired: 2 in]
            n2040 = Array Subset(array=w2501, index=2 ("索引"), length=3 ("长度")) -> (w2510:bool[])
            n2041 = Delete From Array(array=w2500, length=3 ("索引"), index=2 ("长度")) -> (deleted portion=w2511:bool[], array with subset deleted=w2494:bool[])
            n2042 = Array Subset(array=w2504, index=4 ("索引"), length=2 ("长度")) -> (w2509:bool[])
            n2043 = Delete From Array(array=w2530, index=w2529) -> (deleted portion=w2527:refnum<vi>, array with subset deleted=w2528:refnum<vi>[])  [unwired: 1 in]
            n2044 = Insert Into Array(array=w2514, new element #1=w2513, new element #2=w2512, new element #3=w2511, new element #4=w2510, new element #5=w2509, new element #6=w2508) -> (w2507:bool[])  [unwired: 1 in]
            n2045 = Array Subset(array=w2504, index=6 ("索引"), length=2 ("长度")) -> (w2492:bool[])
            n2046 = Array Subset(array=w2501, index=5 ("索引"), length=3 ("长度")) -> (w2493:bool[])
            n2047 = And Array Elements(Boolean array=w2507) -> (logical AND=w2489:bool)
            n2048 = Insert Into Array(array=w2496, new element #1=w2495, new element #2=w2494, new element #3=w2493, new element #4=w2492, new element #5=w2491) -> (w2490:bool[])  [unwired: 1 in]
            n2049 = And Array Elements(Boolean array=w2490) -> (logical AND=w2488:bool)
          }
          frame "单选选项2" {
            n2050 = global read "功能码全局.vi" "18"() -> (w2545:bool[])
            n2051 = global read "功能码全局.vi" "15"() -> (w2566:bool[])
            n2052 = global read "功能码全局.vi" "16"() -> (w2563:bool[])
            n2053 = Delete From Array(array=w2571, index=w2572) -> (deleted portion=w2569:refnum<vi>, array with subset deleted=w2570:refnum<vi>[])  [unwired: 1 in]
            n2054 = Index Array(array=w2563, index #1=4 ("索引"), index #2=5 ("索引"), index #3=6 ("索引"), index #4=7 ("索引")) -> (element #1=w2557:bool, element #2=w2556:bool, element #3=w2552:bool, element #4=w2551:bool)
            n2055 = Index Array(array=w2545, index #1=4 ("索引"), index #2=5 ("索引"), index #3=6 ("索引"), index #4=7 ("索引"), index #5=2 ("索引"), index #6=3 ("索引"), index #7=0 ("索引"), index #8=1 ("索引")) -> (element #1=w2538:bool, element #2=w2541:bool, element #3=w2540:bool, element #4=w2539:bool, element #5=w2537:bool, element #6=w2536:bool, element #7=w2531:bool, element #8=w2532:bool)
            n2056 = Delete From Array(array=w2566, length=4 ("长度"), index=0 ("索引")) -> (deleted portion=w2558:bool[], array with subset deleted=w2553:bool[])
            n2057 = Insert Into Array(array=w2553, new element #1=w2552, new element #2=w2551, new element #3=w2541, new element #4=w2540, new element #5=w2539, new element #6=w2532) -> (w2550:bool[])  [unwired: 1 in]
            n2058 = Insert Into Array(array=w2558, new element #1=w2557, new element #2=w2556, new element #3=w2538, new element #4=w2537, new element #5=w2536, new element #6=w2531) -> (w2555:bool[])  [unwired: 1 in]
            n2059 = And Array Elements(Boolean array=w2555) -> (logical AND=w2554:bool)
            n2060 = And Array Elements(Boolean array=w2550) -> (logical AND=w2549:bool)
          }
        }
        n2061 = property on="全部写入" class="Bool (严格)"("Visible"=w2471) -> ()  [unwired: 2 in, 2 out]
        n2062 = property on="全部读取" class="Bool (严格)"("Visible"=w2470) -> ()  [unwired: 2 in, 2 out]
        n2063 = property on="从板号" class="DigNum (严格)"("Visible"=w2468) -> ()  [unwired: 2 in, 2 out]
        n2064 = local write "主从选择"(w2482) -> ()
        n2065 = property on="从板个数" class="DigNum (严格)"("Visible"=w2474) -> ()  [unwired: 2 in, 2 out]
        n2066 = for {
          tunnel: u32 87470 -> [w2486]
          tunnel: w2479 -> [w2485] mode=indexing
          n2067 = property class="Bool (严格)"(reference=w2485, "BoolText.TextColor"=w2486) -> ()  [unwired: 1 in, 2 out]
        }
        n2068 = Not(x=w2474) -> (.not. x?=w2475:bool)
        n2069 = property class="Bool (严格)"(reference=w2478, "BoolText.TextColor"=u32 16777215) -> ()  [unwired: 1 in, 2 out]
        n2070 = property on="主板选项" class="Tree (严格)"("Visible"=w2474) -> ()  [unwired: 2 in, 2 out]
        n2071 = property on="从板选项" class="Tree (严格)"("Visible"=w2475) -> ()  [unwired: 2 in, 2 out]
        n2072 = property on="当前从板板号" class="DigNum (严格)"("Visible"=w2475) -> ()  [unwired: 2 in, 2 out]
        n2073 = property on="单个读取" class="Bool (严格)"("Visible"=w2469) -> ()  [unwired: 2 in, 2 out]
        n2074 = property on="单个写入" class="Bool (严格)"("Visible"=w2469) -> ()  [unwired: 2 in, 2 out]
      }
      event "从板号": Value Change {
        n2075 = event-data() -> ()  [unwired: 7 out]
        n2076 = local read "key names"() -> (w2574:string[])
        n2077 = Empty Array?(array=w2574) -> (empty?=w2573:bool)
        n2078 = case shown="假" w2573 {
          tunnel: w2574 -> [w2577 _]
          frame False {
            n2079 = stacked-sequence {
              seq-local: [w2578 _] -> [_ w2641]
              tunnel: w2577 -> [w2586 _]
              frame #0 {
                w2617 = 2 ("长度")
                w2614 = 20 ("长度")
                w2602 = 1 ("索引")
                n2080 = local read "从板号"() -> (w2578:u8)
                n2081 = local read "输出数组"() -> (w2587:string[][])
                n2082 = Decrement(x=w2578) -> (x-1=w2584:u8)
                n2083 = Index Array(array=w2587, index (col)=w2584) -> (element=w2615:string[])  [unwired: 1 in]
                n2084 = global write "读配置文件全局2.vi" "从板板号"(w2578) -> ()
                n2085 = Search 1D Array(1D array=w2586, element="风机开启温度" ("元素")) -> (index of element=w2599:i32)  [unwired: 1 in]
                n2086 = Search 1D Array(1D array=w2586, element="电压过高一级" ("元素"), start index (0)=w2599) -> (index of element=w2597:i32)
                n2087 = Decrement(x=w2599) -> (x-1=w2601:i32)
                n2088 = Array Subset(array=w2615, index=w2602, length=w2601) -> (w2585:string[])
                n2089 = Array Subset(array=w2615, index=w2597, length=21 ("长度")) -> (w2589:string[])
                n2090 = Array Subset(array=w2586, index=w2602, length=w2601) -> (w2632:string[])
                n2091 = Array Subset(array=w2615, index=w2599, length=7 ("长度")) -> (w2595:string[])
                n2092 = for {
                  tunnel: w2589 -> [w2634] mode=indexing
                  tunnel: [w2633] -> w2588 mode=indexing
                  n2093 = Fract/Exp String To Number(string=w2634) -> (number=w2633:dbl)  [unwired: 3 in, 1 out]
                }
                n2094 = for {
                  tunnel: w2595 -> [w2636] mode=indexing
                  tunnel: [w2635] -> w2579 mode=indexing
                  n2095 = Fract/Exp String To Number(string=w2636) -> (number=w2635:dbl)  [unwired: 3 in, 1 out]
                }
                n2096 = Delete From Array(array=w2588, length=7 ("长度"), index=0 ("索引")) -> (deleted portion=w2582:dbl[], array with subset deleted=w2592:dbl[])
                n2097 = Array To Cluster(array=w2579) -> (cluster=w2604:T26)
                n2098 = global write "读配置文件全局2.vi" "加热控制参数"(w2579) -> ()
                n2099 = Delete From Array(array=w2592, length=7 ("长度"), index=0 ("索引")) -> (deleted portion=w2581:dbl[], array with subset deleted=w2580:dbl[])
                n2100 = local write "加热控制参数"(w2604) -> ()
                n2101 = Array To Cluster(array=w2582) -> (cluster=w2629:T26)
                n2102 = Array To Cluster(array=w2580) -> (cluster=w2631:T26)
                n2103 = Array To Cluster(array=w2581) -> (cluster=w2630:T26)
                n2104 = global write "读配置文件全局2.vi" "三级故障阀值"(w2580) -> ()
                n2105 = global write "读配置文件全局2.vi" "一级故障阀值"(w2582) -> ()
                n2106 = global write "读配置文件全局2.vi" "二级故障阀值"(w2581) -> ()
                n2107 = local write "一级故障 6"(w2629) -> ()
                n2108 = local write "一级故障 8"(w2631) -> ()
                n2109 = local write "一级故障 7"(w2630) -> ()
                n2110 = Search 1D Array(1D array=w2632, element="温度个数" ("元素")) -> (index of element=w2611:i32)  [unwired: 1 in]
                n2111 = Search 1D Array(1D array=w2632, element="第一个保险通道" ("元素")) -> (index of element=w2612:i32)  [unwired: 1 in]
                n2112 = Search 1D Array(1D array=w2632, element="电压个数" ("元素")) -> (index of element=w2610:i32)  [unwired: 1 in]
                n2113 = Search 1D Array(1D array=w2632, element="第1通道电压个数" ("元素")) -> (index of element=w2613:i32)  [unwired: 1 in]
                n2114 = Array Subset(array=w2585, index=w2610, length=2 ("长度")) -> (w2618:string[])
                n2115 = Array Subset(array=w2585, index=w2611, length=w2617) -> (w2620:string[])
                n2116 = Array Subset(array=w2585, index=w2612, length=20 ("长度")) -> (w2621:string[])
                n2117 = Array Subset(array=w2585, index=w2613, length=w2614) -> (w2619:string[])
                n2118 = Insert Into Array(array=w2618, new element #1=w2619, new element #2=w2620, new element #3=w2621) -> (w2583:string[])  [unwired: 1 in]
                n2119 = Array Subset(array=w2632, index=w2610, length=w2617) -> (w2622:string[])
                n2120 = Array Subset(array=w2632, index=w2611, length=w2617) -> (w2624:string[])
                n2121 = Array Subset(array=w2632, index=w2612, length=w2614) -> (w2625:string[])
                n2122 = Array Subset(array=w2632, index=w2613, length=w2614) -> (w2623:string[])
                n2123 = global write "读配置文件全局2.vi" "表格"(w2583) -> ()
                n2124 = Insert Into Array(array=w2622, new element #1=w2623, new element #2=w2624, new element #3=w2625) -> (w2627:string[])  [unwired: 1 in]
                n2125 = Build Array(w2627, w2583) -> (w2626:string[][])
                n2126 = Transpose 2D Array(2D array=w2626) -> (transposed array=w2628:string[][])
                n2127 = local write "项目信息 2"(w2628) -> ()
              }
              frame #1 {
                n2128 = Number To Decimal String(number=w2641) -> (decimal integer string=w2639:string)  [unwired: 1 in]
                n2129 = control-ref of="结果"() -> (w2644:refnum<vi>)
                n2130 = Concatenate Strings("从板", w2639, "导入完成") -> (w2637:string)
                n2131 = Build Array(w2637) -> (w2642:string[])
                n2132 = call "表格编辑.vi"("新元素/子数组"=w2642, "活动单元格:单元格背景色"=u32 6618880, "MCListbox引用句柄"=w2644) -> ()  [unwired: 9 out]
              }
            }
          }
          frame True {
          }
        }
      }
      event "读配置文件": Value Change {
        n2133 = event-data() -> ("NewVal"=w2645:bool)  [unwired: 6 out]
        n2134 = case shown="真" w2645 {
          tunnel: w2649 -> [w2651 w2657]
          tunnel: [w2651 w2656] -> w2648
          tunnel: w2647 -> [w2650 w2655]
          tunnel: [w2650 w2654] -> w2646
          frame False {
          }
          frame True {
            n2135 = local write "布尔"(TRUE ("布尔")) -> ()
            n2136 = Enqueue Element(queue=w2657, element="读配置文件", error in (no error)=w2655) -> (queue out=w2656:refnum<queue>, error out=w2654:errorcluster)  [unwired: 2 out]
            n2137 = call <vilib>:"Set Busy.vi"() -> ()  [unwired: 4 in, 8 out]
          }
        }
      }
      event "保存主板参数": Value Change {
        n2138 = event-data() -> ("NewVal"=w2658:bool)  [unwired: 6 out]
        n2139 = case shown="真" w2658 {
          tunnel: w2662 -> [w2664 w2669]
          tunnel: [w2664 w2668] -> w2661
          tunnel: w2660 -> [w2663 w2667]
          tunnel: [w2663 w2666] -> w2659
          frame False {
          }
          frame True {
            n2140 = Enqueue Element(queue=w2669, element="写配置文件", error in (no error)=w2667) -> (queue out=w2668:refnum<queue>, error out=w2666:errorcluster)  [unwired: 2 out]
          }
        }
      }
      event "继电器全开": Value Change {
        n2141 = event-data() -> ("NewVal"=w2670:bool)  [unwired: 6 out]
        n2142 = case shown="真" w2670 {
          tunnel: w2670 -> [_ w2673]
          frame False {
          }
          frame True {
            n2143 = stacked-sequence {
              tunnel: w2673 -> [_ w2683 _]
              frame #0 {
                w2674 = FALSE ("清BUFF")
                n2144 = local write "正级继电器"(w2674) -> ()
                n2145 = local write "负级继电器"(w2674) -> ()
                n2146 = local write "充电继电器"(w2674) -> ()
                n2147 = local write "加热继电器"(w2674) -> ()
                n2148 = local write "风机继电器"(w2674) -> ()
                n2149 = local write "预充电继电器"(w2674) -> ()
                n2150 = local write "继电器超时处理"(FALSE ("继电器超时处理")) -> ()
                n2151 = local write "主从选择"(enum32{"主板", "从板"}."主板" ("主从选择")) -> ()
                n2152 = local write "清BUFF"(FALSE ("清BUFF")) -> ()
              }
              frame #1 {
                n2153 = case shown="真" w2683 {
                  selector: w2683 -> [_ w2698]
                  frame False {
                  }
                  frame True {
                    w2694 = 256.0 ("y")
                    w2685 = u32 1 ("命令序号")
                    w2684 = u8 192 ("命令")
                    n2154 = local read "动作保持时间"() -> (w2695:dbl)
                    n2155 = Quotient & Remainder(x=w2695, y=w2694) -> (x-y*floor(x/y)=w2687:dbl, floor(x/y)=w2691:dbl)
                    n2156 = Quotient & Remainder(x=w2691, y=w2694) -> (x-y*floor(x/y)=w2688:dbl, floor(x/y)=w2692:dbl)
                    n2157 = Quotient & Remainder(x=w2692, y=w2694) -> (x-y*floor(x/y)=w2689:dbl, floor(x/y)=w2693:dbl)
                    n2158 = local read "设备索引号"() -> (w2702:u16)
                    n2159 = local read "CAN卡类型"() -> (w2703:u32)
                    n2160 = local read "CAN端口"() -> (w2701:u16)
                    n2161 = Boolean To (0,1)(Boolean=w2698) -> (0, 1=w2696:i16)
                    n2162 = Quotient & Remainder(x=w2693, y=w2694) -> (x-y*floor(x/y)=w2690:dbl)  [unwired: 1 out]
                    n2163 = Build Array(i16 170 ("元素"), w2696, w2690, w2689, w2688, w2687, 0.0 ("元素")) -> (w2699:dbl[])
                    n2164 = call "多帧发送机制(EV05).vi"("can卡类型"=w2703, "设备索引号"=w2702, "CAN端口"=w2701, "命令"=w2684, "板号"=u8 0, "命令序号"=w2685, "输入数据"=w2699) -> ()  [unwired: 1 in, 12 out]
                    n2165 = local write "命令序号"(w2685) -> ()
                    n2166 = local write "命令"(w2684) -> ()
                  }
                }
                n2167 = local write "控制1"(TRUE ("控制1")) -> ()
                n2168 = local write "写?"(FALSE ("写?")) -> ()
                n2169 = local write "消除"(TRUE ("消除")) -> ()
                n2170 = global write "EV05全局变量1.vi" "流控帧 2"(TRUE ("流控帧 2")) -> ()
                n2171 = global write "EV05全局变量1.vi" "流控帧"(FALSE ("流控帧")) -> ()
              }
              frame #2 {
                n2172 = flat-sequence {
                  tunnel: [w2705] -> w2704
                  tunnel: w2704 -> [w2712]
                  frame #0 {
                    n2173 = while {
                      tunnel: [w2706] -> w2705
                      i -> [w2710]
                      stop <- w2707 stop-if-true
                      n2174 = local read "继电器超时处理"() -> (w2706:bool)
                      n2175 = Greater Or Equal?(x=w2710, y=20) -> (x >= y?=w2708:bool)
                      n2176 = Wait Until Next ms Multiple(millisecond multiple=u32 100 ("毫秒倍数")) -> ()  [unwired: 1 out]
                      n2177 = Or(x=w2706, y=w2708) -> (x .or. y?=w2707:bool)
                    }
                  }
                  frame #1 {
                    n2178 = case shown="真" w2712 {
                      frame False {
                        n2179 = One Button Dialog(message="继电器处理超时" ("消息"), button name ("OK")="是" ("按钮名称（“确定”）")) -> ()  [unwired: 1 out]
                      }
                      frame True {
                        w2715 = TRUE ("清BUFF")
                        n2180 = local write "正级继电器"(w2715) -> ()
                        n2181 = local write "负级继电器"(w2715) -> ()
                        n2182 = local write "充电继电器"(w2715) -> ()
                        n2183 = local write "加热继电器"(w2715) -> ()
                        n2184 = local write "风机继电器"(w2715) -> ()
                        n2185 = local write "预充电继电器"(w2715) -> ()
                      }
                    }
                  }
                }
              }
            }
          }
        }
      }
      event "继电器全关": Value Change {
        n2186 = event-data() -> ("NewVal"=w2716:bool)  [unwired: 6 out]
        n2187 = case shown="真" w2716 {
          tunnel: w2716 -> [_ w2719]
          frame False {
          }
          frame True {
            n2188 = stacked-sequence {
              tunnel: w2719 -> [_ w2729 _]
              frame #0 {
                w2720 = TRUE ("清BUFF")
                n2189 = local write "正级继电器"(w2720) -> ()
                n2190 = local write "负级继电器"(w2720) -> ()
                n2191 = local write "充电继电器"(w2720) -> ()
                n2192 = local write "加热继电器"(w2720) -> ()
                n2193 = local write "风机继电器"(w2720) -> ()
                n2194 = local write "预充电继电器"(w2720) -> ()
                n2195 = local write "继电器超时处理"(FALSE ("继电器超时处理")) -> ()
                n2196 = local write "主从选择"(enum32{"主板", "从板"}."主板" ("主从选择")) -> ()
                n2197 = global write "EV05全局变量1.vi" "流控帧"(FALSE ("流控帧")) -> ()
                n2198 = local write "清BUFF"(FALSE ("清BUFF")) -> ()
              }
              frame #1 {
                n2199 = case shown="真" w2729 {
                  selector: w2729 -> [_ w2744]
                  frame False {
                  }
                  frame True {
                    w2740 = 256.0 ("y")
                    w2731 = u32 1 ("命令序号")
                    w2730 = u8 192 ("命令")
                    n2200 = local read "动作保持时间"() -> (w2741:dbl)
                    n2201 = Quotient & Remainder(x=w2741, y=w2740) -> (x-y*floor(x/y)=w2733:dbl, floor(x/y)=w2737:dbl)
                    n2202 = Quotient & Remainder(x=w2737, y=w2740) -> (x-y*floor(x/y)=w2734:dbl, floor(x/y)=w2738:dbl)
                    n2203 = Quotient & Remainder(x=w2738, y=w2740) -> (x-y*floor(x/y)=w2735:dbl, floor(x/y)=w2739:dbl)
                    n2204 = local read "设备索引号"() -> (w2748:u16)
                    n2205 = local read "CAN卡类型"() -> (w2749:u32)
                    n2206 = local read "CAN端口"() -> (w2747:u16)
                    n2207 = Boolean To (0,1)(Boolean=w2744) -> (0, 1=w2742:i16)
                    n2208 = Quotient & Remainder(x=w2739, y=w2740) -> (x-y*floor(x/y)=w2736:dbl)  [unwired: 1 out]
                    n2209 = Build Array(i16 85 ("元素"), w2742, w2736, w2735, w2734, w2733, 0.0 ("元素")) -> (w2745:dbl[])
                    n2210 = call "多帧发送机制(EV05).vi"("can卡类型"=w2749, "设备索引号"=w2748, "CAN端口"=w2747, "命令"=w2730, "板号"=u8 0, "命令序号"=w2731, "输入数据"=w2745) -> ()  [unwired: 1 in, 12 out]
                    n2211 = local write "命令序号"(w2731) -> ()
                    n2212 = local write "命令"(w2730) -> ()
                  }
                }
                n2213 = local write "控制1"(TRUE ("控制1")) -> ()
                n2214 = local write "写?"(FALSE ("写?")) -> ()
                n2215 = local write "消除"(TRUE ("消除")) -> ()
                n2216 = global write "EV05全局变量1.vi" "流控帧 2"(TRUE ("流控帧 2")) -> ()
              }
              frame #2 {
                n2217 = flat-sequence {
                  tunnel: [w2751] -> w2750
                  tunnel: w2750 -> [w2758]
                  frame #0 {
                    n2218 = while {
                      tunnel: [w2752] -> w2751
                      i -> [w2756]
                      stop <- w2753 stop-if-true
                      n2219 = local read "继电器超时处理"() -> (w2752:bool)
                      n2220 = Greater Or Equal?(x=w2756, y=20) -> (x >= y?=w2754:bool)
                      n2221 = Wait Until Next ms Multiple(millisecond multiple=u32 100 ("毫秒倍数")) -> ()  [unwired: 1 out]
                      n2222 = Or(x=w2752, y=w2754) -> (x .or. y?=w2753:bool)
                    }
                  }
                  frame #1 {
                    n2223 = case shown="真" w2758 {
                      frame False {
                        n2224 = One Button Dialog(message="继电器处理超时" ("消息"), button name ("OK")="是" ("按钮名称（“确定”）")) -> ()  [unwired: 1 out]
                      }
                      frame True {
                        w2761 = FALSE ("清BUFF")
                        n2225 = local write "正级继电器"(w2761) -> ()
                        n2226 = local write "负级继电器"(w2761) -> ()
                        n2227 = local write "充电继电器"(w2761) -> ()
                        n2228 = local write "加热继电器"(w2761) -> ()
                        n2229 = local write "风机继电器"(w2761) -> ()
                        n2230 = local write "预充电继电器"(w2761) -> ()
                      }
                    }
                  }
                }
              }
            }
          }
        }
      }
      event "控制按键全为开": Value Change {
        n2231 = event-data() -> ("NewVal"=w2762:bool)  [unwired: 6 out]
        n2232 = case shown="真" w2762 {
          frame False {
          }
          frame True {
            w2763 = TRUE ("正级继电器")
            n2233 = local write "加热继电器(从)"(w2763) -> ()
            n2234 = local write "风机继电器(从)"(w2763) -> ()
            n2235 = local write "DO1 2"(w2763) -> ()
            n2236 = local write "DO1"(w2763) -> ()
            n2237 = local write "DO2"(w2763) -> ()
            n2238 = local write "正级继电器"(w2763) -> ()
            n2239 = local write "负级继电器"(w2763) -> ()
            n2240 = local write "加热继电器"(w2763) -> ()
            n2241 = local write "预充电继电器"(w2763) -> ()
            n2242 = local write "充电继电器"(w2763) -> ()
            n2243 = local write "风机继电器"(w2763) -> ()
          }
        }
      }
      event "控制按键全为关": Value Change {
        n2244 = event-data() -> ("NewVal"=w2764:bool)  [unwired: 6 out]
        n2245 = case shown="真" w2764 {
          frame False {
          }
          frame True {
            w2765 = FALSE ("正级继电器")
            n2246 = local write "加热继电器(从)"(w2765) -> ()
            n2247 = local write "风机继电器(从)"(w2765) -> ()
            n2248 = local write "DO1 2"(w2765) -> ()
            n2249 = local write "DO1"(w2765) -> ()
            n2250 = local write "DO2"(w2765) -> ()
            n2251 = local write "正级继电器"(w2765) -> ()
            n2252 = local write "负级继电器"(w2765) -> ()
            n2253 = local write "加热继电器"(w2765) -> ()
            n2254 = local write "预充电继电器"(w2765) -> ()
            n2255 = local write "充电继电器"(w2765) -> ()
            n2256 = local write "风机继电器"(w2765) -> ()
          }
        }
      }
      event "正级继电器": Value Change {
        n2257 = event-data() -> ("NewVal"=w2766:bool)  [unwired: 6 out]
        n2258 = stacked-sequence {
          tunnel: w2766 -> [_ w2779 _]
          frame #0 {
            w2769 = FALSE ("清BUFF")
            n2259 = local write "继电器超时处理"(FALSE ("继电器超时处理")) -> ()
            n2260 = local write "主从选择"(enum32{"主板", "从板"}."主板" ("主从选择")) -> ()
            n2261 = local write "正级继电器 12"(w2769) -> ()
            n2262 = local write "清BUFF"(w2769) -> ()
          }
          frame #1 {
            n2263 = case shown="假" w2779 {
              selector: w2779 -> [w2794 w2814]
              tunnel: [w2793 w2813] -> w2778
              tunnel: [w2781 w2801] -> w2773
              frame False {
                w2789 = 256.0 ("y")
                w2781 = u32 1 ("命令序号")
                w2793 = u8 192 ("命令")
                n2264 = local read "动作保持时间"() -> (w2790:dbl)
                n2265 = Quotient & Remainder(x=w2790, y=w2789) -> (x-y*floor(x/y)=w2782:dbl, floor(x/y)=w2786:dbl)
                n2266 = Quotient & Remainder(x=w2786, y=w2789) -> (x-y*floor(x/y)=w2783:dbl, floor(x/y)=w2787:dbl)
                n2267 = Quotient & Remainder(x=w2787, y=w2789) -> (x-y*floor(x/y)=w2784:dbl, floor(x/y)=w2788:dbl)
